vi "Test Panel.vi"() -> ()   [LabVIEW 2020]
doc: "This example performs writes and reads on a serial port, as directed by the user. You can press the Write and Read buttons, and change the Read Count, while the example is running.\n\nThe parameters set for the serial port must match the parameters of the connected instrument or device. In this example, the Read Count parameter specifies the number of bytes that the serial port reads. If there were more bytes at the port than the specified number, those bytes would not be read. If there were less bytes at the port than the specified number, you would receive a timeout error.\n\nThis example expands upon the flow control options for XON and XOFF, allowing the user to choose those control characters. Also, the user can enable or disable a termination character. Some devices require a termination character in order to identify the end of command strings. Some devices send a termination character to signify the end of data to be read. This example shows how you can end the Read operation once a termination character is detected in the buffer and/or append a termination character at the end of the Write data."
uses:
  <extravilib>/ChannelInstances/Tag-bool/Write With Abort.vi
  <extravilib>/ChannelInstances/Tag-bool/Read With Abort.vi
  <extravilib>/ChannelInstances/Tag-bool/Instantiate.vi
  <extravilib>/ChannelInstances/Tag-bool/EndpointRead.vi
  <instrlib>/BDAQ-6104/Public/Data/Stop Streaming.vi
  <instrlib>/BDAQ-6104/Public/Data/Start Streaming.vi
  <extravilib>/ChannelInstances/Tag-bool/Endpoint.vi
  <extravilib>/ChannelInstances/Tag-bool.lvlib
  <instrlib>/BDAQ-6104/BDAQ-6104.lvlib
panel:
  out "Digital Inputs":T1
  in  "Samples per Second":i32=100 min=1 max=1000
  in  "VISA resource name":refnum<visa-resource-name>
  in  "Voltage Data":bool=TRUE
  out "Anolog Input Channels":T2(graph)
  in  "stop":bool
  in  "Stream Data":bool
  # "Raw Data"
  # "The Test Panel runs the DAQ module in streaming mode allowing the user to test both the Digital and Analog input functions.\nA sample rate between 1 to 1000 samples per second can be specified."
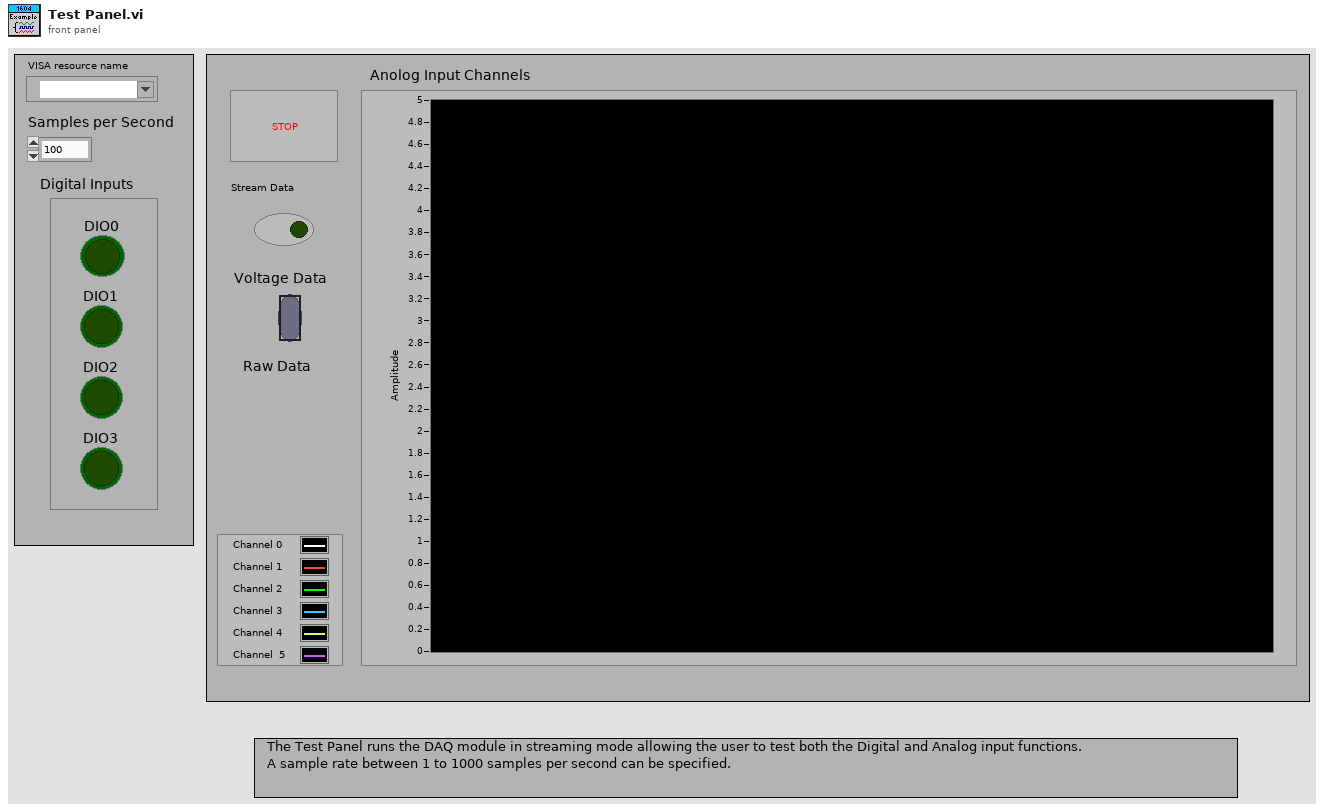
[diagram p1: front panel]
types:
  T1 = cluster{"DIO0":bool, "DIO2":bool, "DIO3":bool, "DIO1":bool}
  T2 = cluster{"AIO-0":dbl, "AIO-1":dbl, "AIO-2":dbl, "AIO-3":dbl, "AIO-4":dbl, "AIO-5":dbl}
  T3 = cluster{"AIO-0":dbl, "AIO-1":dbl, "AIO-2":dbl, "AIO-3":dbl, "AIO-4":dbl, "AIO-5":dbl}[]
  T4 = typedef "Tag-bool.lvlib/))Channel.ctl" = refnum<queue>
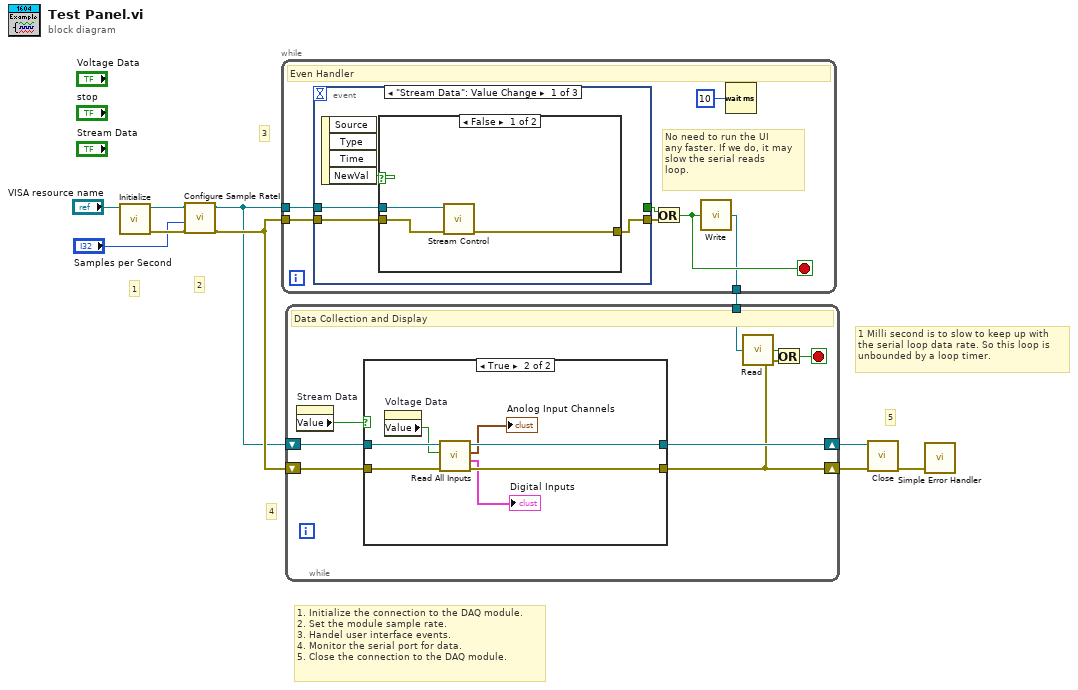
[diagram p0: block diagram]
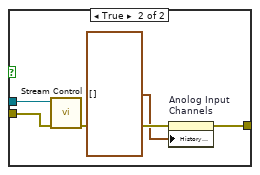
[diagram p3: hidden frame]
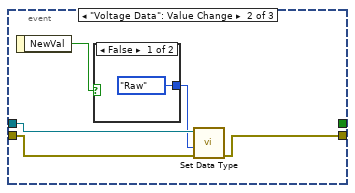
[diagram p4: hidden frame]
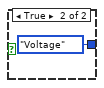
[diagram p5: hidden frame]
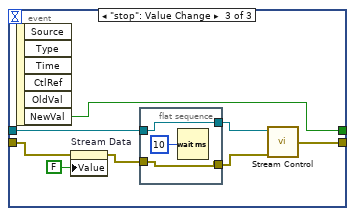
[diagram p6: hidden frame]
diagram:
  # "1. Initialize the connection to the DAQ module.\n2. Set the module sample rate.\n3. Handel user interface events.\n4. Monitor the serial port for data.\n5. Close the connection to the DAQ module."
  # "5"
  # "4"
  # "3"
  # "2"
  # "1"
  # "1 Milli second is to slow to keep up with\nthe serial loop data rate. So this loop is\nunbounded by a loop timer."
  n1 = call <instrlib>:"Initialize.vi"("VISA resource name"="VISA resource name") -> ("error out"=w5:errorcluster, "VISA resource name out"=w6:refnum<visa-resource-name>)  [unwired: 9 in]
  n2 = call <instrlib>:"Configure Sample RateI.vi"("error in"=w5, "Samples per Second"="Samples per Second", "VISA resource name"=w6) -> ("error out"=w8:errorcluster, "VISA resource name out"=w7:refnum<visa-resource-name>)  [unwired: 7 in]
  n3 = while {
    tunnel: w8 -> [w16]
    tunnel: w7 -> [w13]
    tunnel: [w11] -> w10
    stop <- w12 stop-if-true
    # "No need to run the UI\nany faster. If we do, it may\nslow the serial reads\nloop."
    # "Even Handler"
    n4 = event shown="[0] \"Stream Data\": Value Change" {
      selector: _ -> [_ _ _]
      dyn-events: _ -> [_ _ _]
      timeout: _ -> [_ _ _]
      tunnel: w13 -> [w20 w33 w38]
      tunnel: [w18 w30 w43] -> w15
      tunnel: w16 -> [w19 w32 w42]
      tunnel: [_ _ w44] -> w14
      event "Stream Data": Value Change {
        n5 = event-data() -> ("NewVal"=w21:bool)  [unwired: 1 in, 3 out]
        n6 = case shown="False" w21 {
          tunnel: w20 -> [w24 w29]
          tunnel: w19 -> [w23 w28]
          tunnel: [w22 w26] -> w18
          frame False {
            n7 = call-poly <instrlib>:"Stream Control.vi"("error in (no error)"=w23, "VISA resource name"=w24) -> ("error out"=w22:errorcluster)  [unwired: 8 in, 1 out]
          }
          frame True {
            n8 = call-poly <instrlib>:"Stream Control.vi"("error in (no error)"=w28, "VISA resource name"=w29) -> ("error out"=w27:errorcluster)  [unwired: 8 in, 1 out]
            n9 = property on="Anolog Input \nChannels" class="WFChart (strict)"(error in=w27, "History Data"=T3 []) -> (error out=w26:errorcluster)  [unwired: 1 in, 1 out]
          }
        }
      }
      event "Voltage Data": Value Change {
        n10 = event-data() -> ("NewVal"=w34:bool)  [unwired: 1 in]
        n11 = case shown="False" w34 {
          tunnel: [enum16{"Voltage", "Raw"}."Raw" ("Data Type") enum16{"Voltage", "Raw"}."Voltage" ("Data Type")] -> w31
          frame False {
          }
          frame True {
          }
        }
        n12 = call <instrlib>:"Set Data Type.vi"("error in (no error)"=w32, "Data Type"=w31, "VISA resource name"=w33) -> ("error out"=w30:errorcluster)  [unwired: 7 in, 1 out]
      }
      event "stop": Value Change {
        n13 = event-data() -> ("NewVal"=w44:bool)  [unwired: 1 in, 5 out]
        n14 = property on="Stream Data" class="Bool (strict)"(error in=w42, "Value"=FALSE ("Stream Data")) -> (error out=w40:errorcluster)  [unwired: 1 in, 1 out]
        n15 = flat-sequence {
          tunnel: w40 -> [w46]
          tunnel: [w46] -> w39
          tunnel: w38 -> [w45]
          tunnel: [w45] -> w37
          frame #0 {
            n16 = Wait (ms)(milliseconds to wait=u32 10) -> ()  [unwired: 1 out]
          }
        }
        n17 = call-poly <instrlib>:"Stream Control.vi"("error in (no error)"=w39, "VISA resource name"=w37) -> ("error out"=w43:errorcluster)  [unwired: 8 in, 1 out]
      }
    }
    n18 = Or(x=w14, y=w15) -> (x .or. y?=w12:bool)
    n19 = call <extravilib>:"Write.vi"("element"=w12) -> ("channel"=w11:T4)  [unwired: 1 out]
    n20 = Wait (ms)(milliseconds to wait=u32 10) -> ()  [unwired: 1 out]
  }
  n21 = while {
    shift-right: [w49] -> w3
    shift-left: w8 -> [w53]
    shift-right: [w54] -> w1
    shift-left: w7 -> [w55]
    tunnel: w10 -> [w52]
    stop <- w48 stop-if-true
    # "Data Collection and Display"
    n22 = property on="Stream Data" class="Bool (strict)"() -> ("Value"=w51:bool)  [unwired: 2 in, 2 out]
    n23 = case shown="True" w51 {
      tunnel: w55 -> [w57 w64]
      tunnel: [w57 w61] -> w54
      tunnel: [w56 w62] -> w49
      tunnel: w53 -> [w56 w63]
      frame False {
      }
      frame True {
        n24 = property on="Voltage Data" class="Bool (strict)"() -> ("Value"=w60:bool)  [unwired: 2 in, 2 out]
        n25 = call <instrlib>:"Read All Inputs.vi"("error in"=w63, "Voltage"=w60, "VISA resource name"=w64) -> ("error out"=w62:errorcluster, "Digital Output cluster"=→"Digital Inputs":T1, "Analog output cluster"=→"Anolog Input Channels":T2, "VISA resource name out"=w61:refnum<visa-resource-name>)  [unwired: 5 in]
      }
    }
    n26 = call <extravilib>:"Read.vi"("channel"=w52) -> ("element"=w50:bool)  [unwired: 1 in, 1 out]
    n27 = Or(x=w50, y=w49) -> (x .or. y?=w48:bool)
  }
  n28 = call <instrlib>:"Close.vi"("error in (no error)"=w3, "VISA resource name"=w1) -> ("error out"=w2:errorcluster)  [unwired: 9 in]
  n29 = call <vilib>:"Simple Error Handler.vi"("error in (no error)"=w2) -> ()  [unwired: 1 in, 8 out]
